vi "Extract LVCLASS-Taged Classname.vi"(1 "Tagged LVClass Name":string) -> (0 "found?":bool, 2 "LVClass Name":string)   [LabVIEW 2014, in "CS++Utilities.lvlib"]
doc: "Extract classname from tagged string <LVCLASS>classname</LVCLASS>."
uses:
  CS++Utilities.lvlib
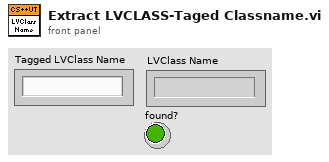
[diagram p1: front panel]
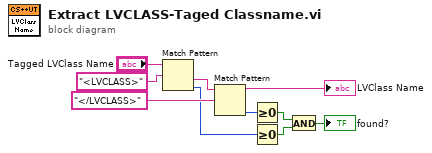
[diagram p0: block diagram]
diagram:
  n1 = Match Pattern(string="Tagged LVClass Name", regular expression="<LVCLASS>" ("string")) -> (after substring=w10:string, offset past match=w5:i32)  [unwired: 1 in, 2 out]
  n2 = Match Pattern(string=w10, regular expression="</LVCLASS>" ("string")) -> (before substring=→"LVClass Name":string, offset past match=w4:i32)  [unwired: 1 in, 2 out]
  n3 = Greater Or Equal To 0?(x=w4) -> (x >= 0?=w3:bool)
  n4 = Greater Or Equal To 0?(x=w5) -> (x >= 0?=w2:bool)
  n5 = And(x=w3, y=w2) -> (x .and. y?=→"found?":bool)
